vi "Ultrasonic Data.vi"() -> ()   [LabVIEW 2014]
panel:
  in  "Right":dbl
  in  "Left":dbl
  in  "Back":dbl
  in  "Front":dbl
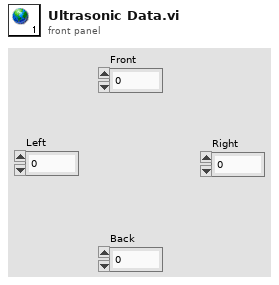
[diagram p1: front panel]
diagram:
